vi "Remove Processor.vi"(8 "error in (no error)":errorcluster, 10 "Label":string, 11 "ImagePipeline in":refnum<class "ImagePipeline.lvclass">) -> (0 "error out":errorcluster, 3 "ImagePipeline out":refnum<class "ImagePipeline.lvclass">)   [LabVIEW 2020, in "ImagePipeline.lvlib" / "ImagePipeline.lvclass"]
uses:
  ImagePipeline.lvclass
  ImagePipeline.lvclass/ImagePipeline.ctl
  <vilib>/ActorFramework/Message Enqueuer/Message Enqueuer.lvclass/Message Enqueuer.ctl
  <vilib>/ActorFramework/Message Enqueuer/Enqueue.vi
  <vilib>/ActorFramework/Stop Msg/Stop Msg.lvclass
  C:/Program Files/National Instruments/LabVIEW 2020/vi.lib/ActorFramework/Message/Message.lvclass
  <vilib>/ActorFramework/Message Priority Queue/Priority Enqueue.vi
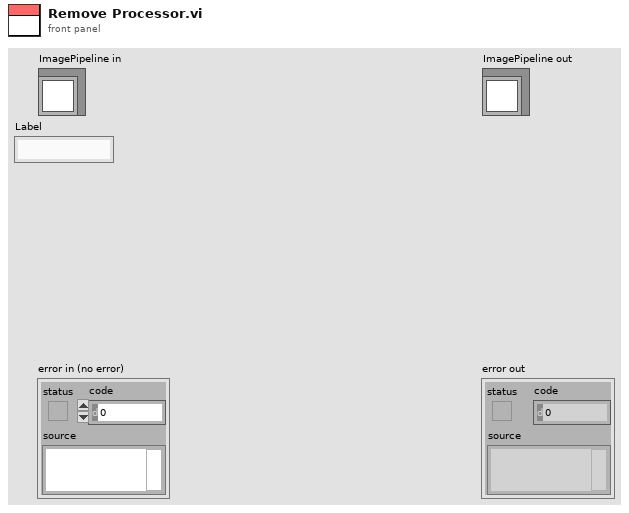
[diagram p1: front panel]
types:
  T1 = map{string, refnum<class "Message Enqueuer.lvclass">}
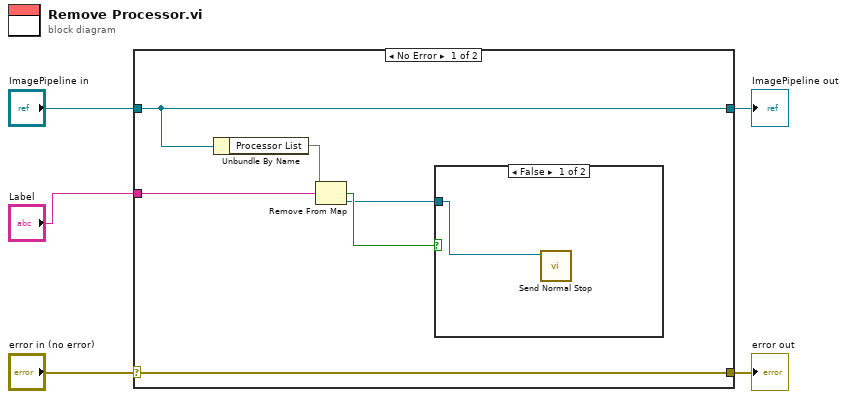
[diagram p0: block diagram]
diagram:
  n1 = case shown="No Error" "error in (no error)" {
    selector: "error in (no error)" -> [w11 w14]
    tunnel: [w11 w14] -> w4
    tunnel: [w10 w13] -> w2
    tunnel: "ImagePipeline in" -> [w10 w13]
    tunnel: "Label" -> [w8 _]
    frame No Error {
      n2 = Unbundle By Name(w10) -> ("Processor List"=w9:T1)
      n3 = Remove From Map(10:w8, 11:w9) -> (1:w6:refnum<class "Message Enqueuer.lvclass">, 2:w7:bool)  [unwired: 1 out]
      n4 = case shown="False" w7 {
        tunnel: w6 -> [w12 _]
        frame False {
          n5 = call <vilib>:"Send Normal Stop.vi"("Message Enqueuer"=w12) -> ()  [unwired: 10 in, 1 out]
        }
        frame True {
        }
      }
    }
    frame Error {
    }
  }
  "error out" <- w4
  "ImagePipeline out" <- w2
